vi "Get IO Config Path.vi"(8 "error in (no error)":errorcluster) -> (0 "error out":errorcluster, 1 "DO COnfig path":path, 2 "DI Config path":path, 3 "AO Config path":path, 4 "Limit Path":T1, 5 "AI Config path":path)   [LabVIEW 2025]
uses:
  Controls/Limit Paths.ctl
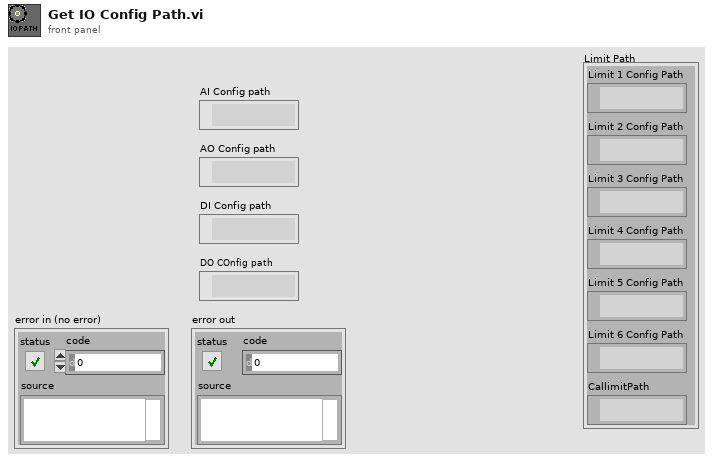
[diagram p1: front panel]
types:
  T1 = typedef "Limit Paths.ctl" = cluster{"Limit 1 Config Path":path, "Limit 2 Config Path ":path, "Limit 3 Config Path ":path, "Limit 4 Config Path ":path, "Limit 5 Config Path ":path, "Limit 6 Config Path ":path, "CallimitPath ":path}
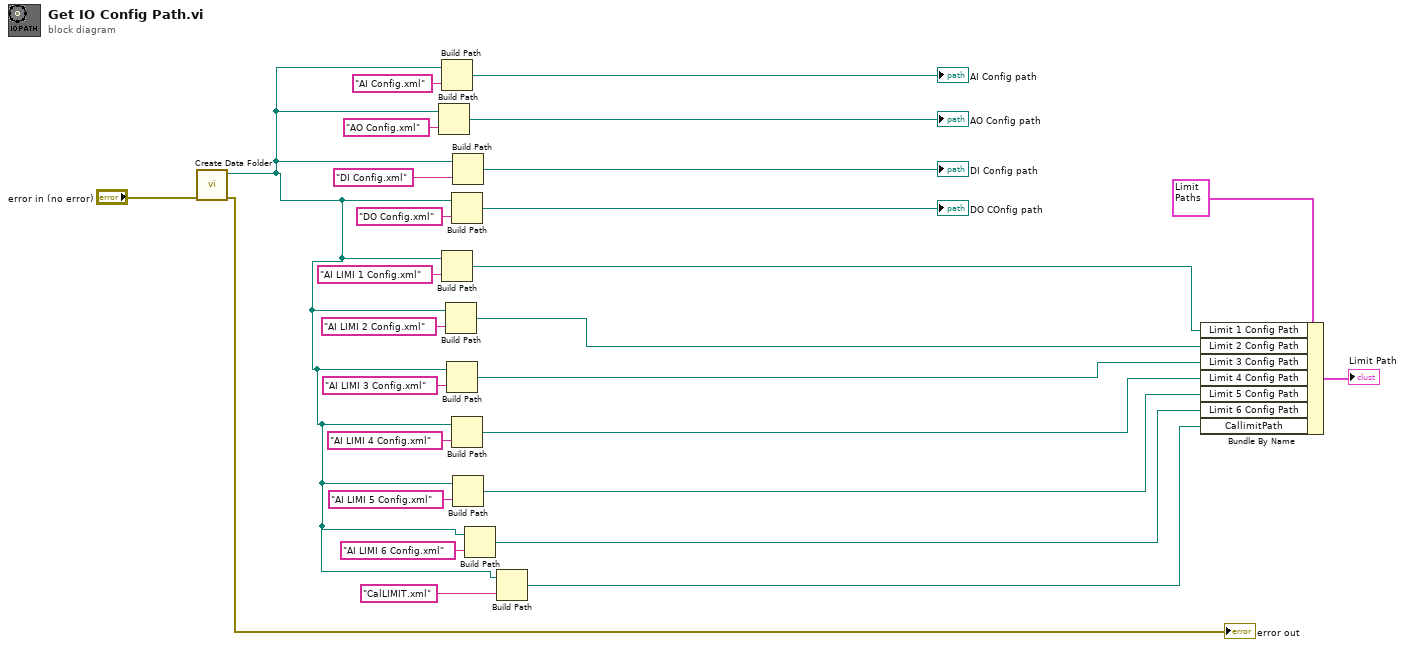
[diagram p0: block diagram]
diagram:
  n1 = call "Create Data Folder.vi"("error in (no error)"="error in (no error)") -> ("error out"=→"error out":errorcluster, "Data path"=w2:path)  [unwired: 9 in]
  n2 = Build Path(base path=w2, name or relative path="AO Config.xml") -> (appended path=→"AO Config path":path)
  n3 = Build Path(base path=w2, name or relative path="AI Config.xml") -> (appended path=→"AI Config path":path)
  n4 = Build Path(base path=w2, name or relative path="AI LIMI 1 Config.xml") -> (appended path=w11:path)
  n5 = Build Path(base path=w2, name or relative path="AI LIMI 2 Config.xml") -> (appended path=w10:path)
  n6 = Build Path(base path=w2, name or relative path="AI LIMI 3 Config.xml") -> (appended path=w9:path)
  n7 = Build Path(base path=w2, name or relative path="DO Config.xml") -> (appended path=→"DO COnfig path":path)
  n8 = Build Path(base path=w2, name or relative path="AI LIMI 4 Config.xml") -> (appended path=w8:path)
  n9 = Build Path(base path=w2, name or relative path="DI Config.xml") -> (appended path=→"DI Config path":path)
  n10 = Build Path(base path=w2, name or relative path="AI LIMI 5 Config.xml") -> (appended path=w7:path)
  n11 = Build Path(base path=w2, name or relative path="AI LIMI 6 Config.xml") -> (appended path=w6:path)
  n12 = Build Path(base path=w2, name or relative path="CalLIMIT.xml") -> (appended path=w1:path)
  n13 = Bundle By Name(cluster=T1 {"Limit 1 Config Path"=path "", "Limit 2 Config Path "=path "", "Limit 3 Config Path "=path "", "Limit 4 Config Path "=path "", "Limit 5 Config Path "=path "", "Limit 6 Config Path "=path "", "CallimitPath "=path ""} ("Limit Path"), "Limit 1 Config Path"=w11, "Limit 2 Config Path"=w10, "Limit 3 Config Path"=w9, "Limit 4 Config Path"=w8, "Limit 5 Config Path"=w7, "Limit 6 Config Path"=w6, "CallimitPath"=w1) -> (→"Limit Path":T1)
